vi "Read allow debugging.vi"(8 "error in (no error)":errorcluster, 11 "execution settings in":refnum<class "execution settings.lvclass">) -> (0 "error out":errorcluster, 2 "allow debugging":bool, 3 "execution settings out":refnum<class "execution settings.lvclass">)   [LabVIEW 2013, in "execution settings.lvclass"]
uses:
  execution settings.lvclass
  execution settings.lvclass/execution settings.ctl
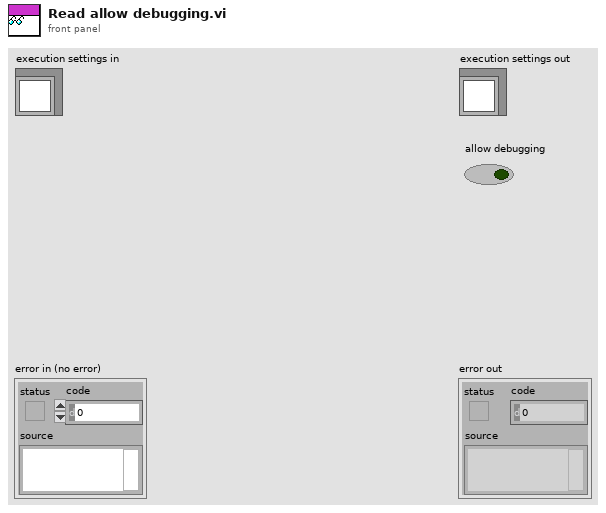
[diagram p1: front panel]
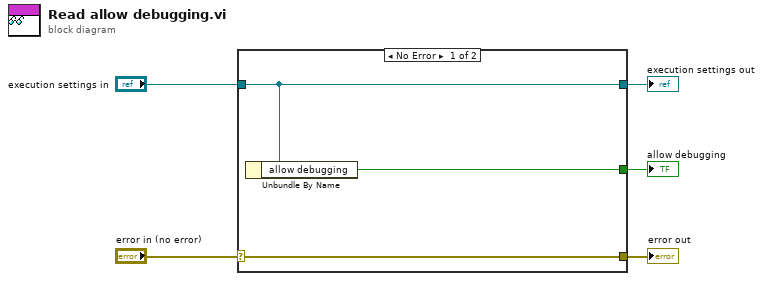
[diagram p0: block diagram]
diagram:
  n1 = case shown="No Error" "error in (no error)" {
    selector: "error in (no error)" -> [w8 w9]
    tunnel: [w8 w9] -> w4
    tunnel: [w7 w10] -> w2
    tunnel: "execution settings in" -> [w7 w10]
    tunnel: [w6 _] -> w1
    frame No Error {
      n2 = Unbundle By Name(w7) -> ("allow debugging"=w6:bool)
    }
    frame Error {
    }
  }
  "error out" <- w4
  "execution settings out" <- w2
  "allow debugging" <- w1
